vi "Renishaw-XL80_CancelPreHeat.vi"(8 "error in (no error)":errorcluster, 11 "Renishaw-XL80_EMU in":refnum<class "Renishaw-XL80_EMU.lvclass">) -> (0 "error out":errorcluster, 3 "Renishaw-XL80_EMU out":refnum<class "Renishaw-XL80_EMU.lvclass">)   [LabVIEW 2024, in "Renishaw-XL80_EMU.lvclass"]
doc: "This method will terminate the preheat cycle of the ML10. This method should be used with caution, since shortening the preheat cycle may lead to loss of laser stability later.\n\nDefinition\nHRESULTCancelPreheat();\nParameters\nNone\n\nComments\nThis method will return with an HRESULT of E_FAIL if the client has not previously connected to a DX10 by calling Connect. The method will also return E_FAIL if the DX10 is not responding or the ML10 is not responding.\n\nIf the method is successful it will return with an HESULT of S_OK.\n\nNote that this method succeeds even if the ML10 was not in a preheat cycle."
uses:
  Renishaw-XL80_EMU.lvclass
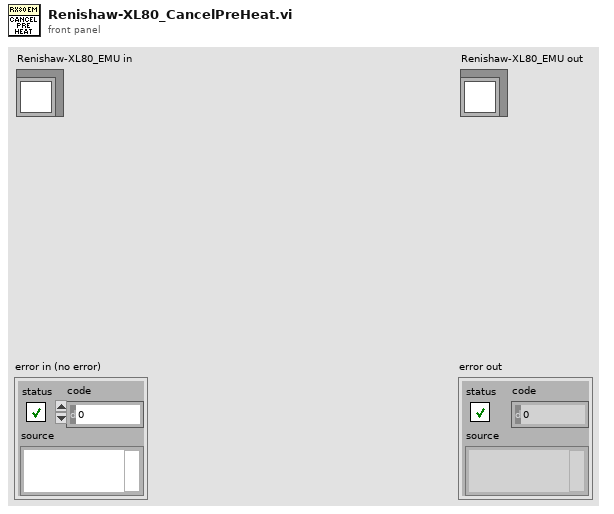
[diagram p1: front panel]
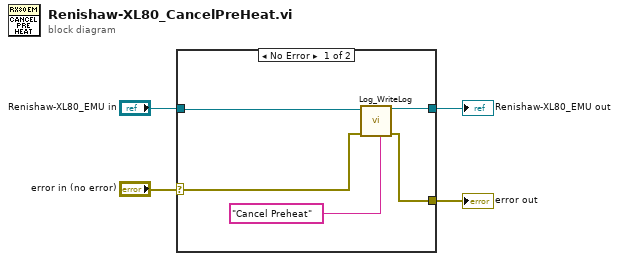
[diagram p0: block diagram]
diagram:
  n1 = case shown="No Error" "error in (no error)" {
    selector: "error in (no error)" -> [w5 w11]
    tunnel: [w7 w11] -> w1
    tunnel: [w8 w10] -> w2
    tunnel: "Renishaw-XL80_EMU in" -> [w6 w10]
    frame No Error {
      n2 = call-dynamic "Log_WriteLog.vi"("Additional text"="Cancel Preheat", "error in (no error)"=w5, "Log in"=w6) -> ("error out"=w7:errorcluster, "Log out"=w8:refnum<class "Renishaw-XL80_EMU.lvclass">)  [unwired: 7 in]
    }
    frame Error {
    }
  }
  "error out" <- w1
  "Renishaw-XL80_EMU out" <- w2
